vi "mcc_usb202_open.vi"(6 "error in":errorcluster, 11 "name":string="Dev1/Ai0:1") -> (0 "status":bool=TRUE, 3 "task out":refnum<k24>, 4 "error out":errorcluster={"status"=TRUE, "code"=10023, "source"="ULx Create Channel (AI-Voltage-Basic).vi:5780001<ERR>\nMeasurements: Channel not specified."})   [LabVIEW 2019]
uses:
  C:/Program Files/National Instruments/LabVIEW 2019/vi.lib/ULx/ULx_LV.dll
  Program Files/National Instruments/LabVIEW 2019/vi.lib/ULx/ULx_LV.dll
  <vilib>/ULx/Create Channel.llb/ULx Create Channel (AI-Voltage-Basic).vi
  <vilib>/ULx/Timing.llb/ULx Timing (Sample Clock).vi
panel:
  in  "samples per channel":i32=500
  in  "Refnum":refnum<k21>
  # "\"Refnum\" is used only to find available devices."
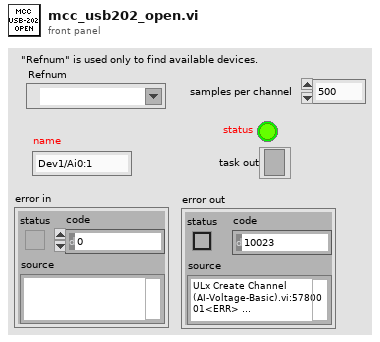
[diagram p1: front panel]
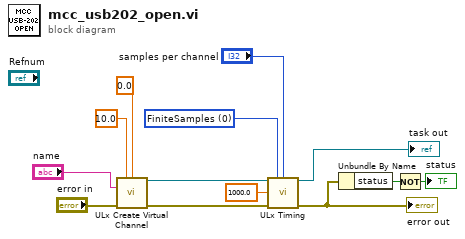
[diagram p0: block diagram]
diagram:
  w8 = 0 items=["FiniteSamples", "ContinuousSamples"] ("Sampling Mode")
  n1 = call-poly <vilib>:"ULx Create Virtual Channel.vi"("maximum value"=10.0 ("Max Value"), "minimum value"=0.0 ("Min Value"), "physical channels"="name", "error in"="error in") -> ("task out"=w9:refnum<k24>, "error out"=w10:errorcluster)  [unwired: 10 in]
  n2 = call-poly <vilib>:"ULx Timing.vi"("task in"=w9, "sample mode"=w8, "samples per channel"="samples per channel", "rate"=1000.0, "error in"=w10) -> ("task out"=→"task out":refnum<k24>, "error out"=w4:errorcluster)  [unwired: 9 in]
  "error out" <- w4
  n3 = Unbundle By Name(w4) -> ("status"=w1:bool)
  n4 = Not(x=w1) -> (.not. x?=→"status":bool)
